vi "Initialize.vi"(7 "Serial Configuration":T1={"Baud Rate"=19200, "Parity"=0, "Data Bits"=8, "Stop Bits"=10, "Flow Control"=2} {"Flow Control" items=["None"=0, "RTS/CTS"=2]; "Stop Bits" items=["1.0"=10]; "Data Bits" items=["8"=8]; "Parity" items=["None"]; "Baud Rate" items=["9600"=9600, "19200"=19200, "38400"=38400]}, 8 "error in (no error)":errorcluster, 9 "Reset (True)":bool=TRUE, 10 "ID Query (True)":bool=TRUE, 11 "VISA resource name":refnum<visa-resource-name>) -> (0 "error out":errorcluster, 3 "VISA resource name out":refnum<visa-resource-name>)   [LabVIEW 2015, in "Voltech PM1000+.lvlib"]
doc: "Establishes communication with the instrument and optionally performs an instrument identification query and/or an instrument reset. It also places the instrument in a default state needed for other instrument driver operations. Therefore, call this VI before calling other instrument driver VIs for this instrument. Generally, you need to call the Initialize VI only once at the beginning of an application."
uses:
  <instrlib>/Voltech PM1000+/Voltech PM1000+.lvlib
panel:
  # "(c) 2008-2009 Voltech Instruments.  ALL RIGHTS RESERVED."
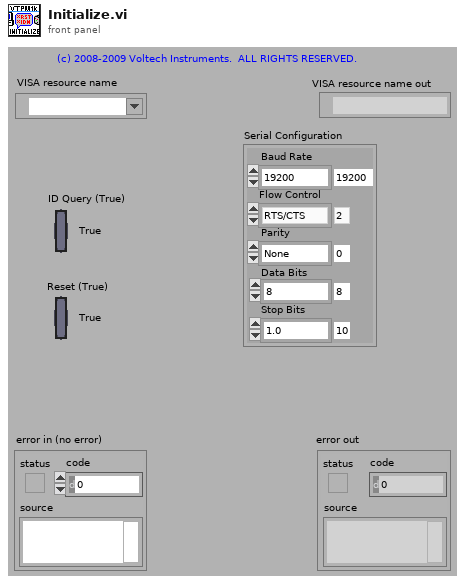
[diagram p1: front panel]
types:
  T1 = cluster{"Baud Rate":u32, "Parity":u16, "Data Bits":u16, "Stop Bits":u16, "Flow Control":u16}
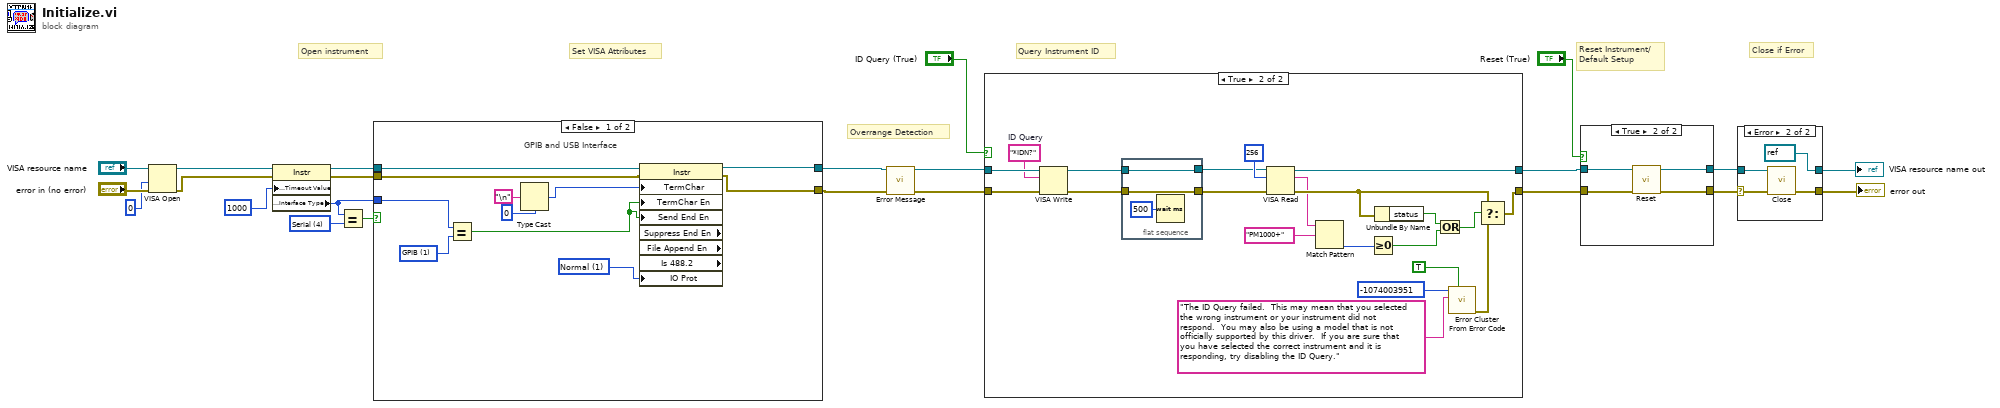
[diagram p0: block diagram]
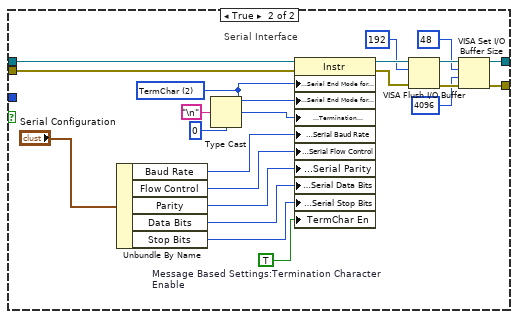
[diagram p2: hidden frame]
diagram:
  w15 = u16 4 items=["GPIB"=1, "Serial"=4, "USB"=7] ("Interface Information:Interface Type")
  # "Overrange Detection"
  # "Set VISA Attributes"
  # "Close if Error"
  # "Query Instrument ID"
  # "Reset Instrument/\nDefault Setup"
  # "Open instrument"
  n1 = VISA Open(access mode=u32 0, error in (no error)="error in (no error)", VISA resource name="VISA resource name") -> (VISA resource name=w8:refnum<visa-resource-name>, error out=w7:errorcluster)  [unwired: 2 in]
  n2 = property class="Instr"(reference=w8, error in=w7, "General Settings:Timeout Value"=u32 1000) -> (reference out=w18:refnum<visa-resource-name>, error out=w17:errorcluster, "Interface Information:Interface Type"=w9:u16)
  n3 = Equal?(x=w9, y=w15) -> (x = y?=w16:bool)
  n4 = case shown="False" w16 {
    tunnel: [w32 w53] -> w6
    tunnel: [w31 w50] -> w3
    tunnel: w18 -> [w34 w55]
    tunnel: w17 -> [w33 w56]
    tunnel: w9 -> [w25 _]
    frame False {
      w26 = u16 1 items=["GPIB"=1, "Serial"=4, "USB"=7] ("Interface Information:Interface Type")
      w27 = u16 1 items=["Normal"=1, "VXI/FDC"=2, "GPIB/HS488"=3, "Serial-TCPIP-USB/488 Strings"=4, "USBTMC/Vendor-Specific"=5] ("Message Based Settings:IO Protocol")
      # "GPIB and USB Interface"
      n5 = Equal?(x=w25, y=w26) -> (x = y?=w24:bool)
      n6 = Type Cast(type=u8 0, x="\n" ("Line Feed Constant")) -> (*(type *) &x=w28:u8)
      n7 = property class="Instr" props=["TermChar", "TermChar En", "Send End En", "Suppress End En", "File Append En", "Is 488.2", "IO Prot"](reference=w34, error in=w33, "TermChar"=w28, "TermChar En"=w24, "Send End En"=w24, "IO Prot"=w27) -> (reference out=w32:refnum<visa-resource-name>, error out=w31:errorcluster)  [unwired: 3 out]
    }
    frame True {
      w43 = u16 2 items=["None", "LastBit", "TermChar"] ("Serial Settings:Serial End Mode for Reads")
      w35 = TRUE  # Message Based Settings:Termination Character Enable
      # "Serial Interface"
      n8 = Unbundle By Name("Serial Configuration") -> ("Baud Rate"=w41:u32, "Flow Control"=w37:u16, "Parity"=w39:u16, "Data Bits"=w40:u16, "Stop Bits"=w36:u16)
      n9 = Type Cast(type=u8 0, x="\n" ("Line Feed Constant")) -> (*(type *) &x=w42:u8)
      n10 = property class="Instr"(reference=w55, error in=w56, "Serial Settings:Serial End Mode for Reads"=w43, "Serial Settings:Serial End Mode for Writes"=w43, "Message Based Settings:Termination Character"=w42, "Serial Settings:Serial Baud Rate"=w41, "Serial Settings:Serial Flow Control"=w37, "Serial Settings:Serial Parity"=w39, "Serial Settings:Serial Data Bits"=w40, "Serial Settings:Serial Stop Bits"=w36, "TermChar En"=w35) -> (reference out=w49:refnum<visa-resource-name>, error out=w52:errorcluster)
      n11 = VISA Flush I/O Buffer(VISA resource name=w49, mask (16)=u16 192, error in (no error)=w52) -> (VISA resource name out=w54:refnum<visa-resource-name>, error out=w51:errorcluster)
      n12 = VISA Set I/O Buffer Size(VISA resource name=w54, mask (16)=u16 48, size (4096)=u32 4096 ("size (0)"), error in (no error)=w51) -> (VISA resource name out=w53:refnum<visa-resource-name>, error out=w50:errorcluster)
    }
  }
  n13 = call <instrlib>:"Error Message.vi"("VISA resource name"=w6, "error in (no error)"=w3) -> ("VISA resource name out"=w4:refnum<visa-resource-name>, "error out"=w5:errorcluster)  [unwired: 12 in]
  n14 = case shown="True" "ID Query (True)" {
    tunnel: [w57 w79] -> w1
    tunnel: [w58 w76] -> w2
    tunnel: w4 -> [w58 w77]
    tunnel: w5 -> [w57 w78]
    frame False {
    }
    frame True {
      w73 = "*IDN?"  # ID Query
      n15 = VISA Write(VISA resource name=w77, write buffer=w73, error in (no error)=w78) -> (VISA resource name out=w62:refnum<visa-resource-name>, error out=w60:errorcluster)  [unwired: 1 out]
      n16 = flat-sequence {
        tunnel: [w81] -> w61
        tunnel: w62 -> [w81]
        tunnel: [w80] -> w59
        tunnel: w60 -> [w80]
        frame #0 {
          n17 = Wait (ms)(milliseconds to wait=500) -> ()  [unwired: 1 out]
        }
      }
      n18 = VISA Read(VISA resource name=w61, byte count=u32 256, error in (no error)=w59) -> (VISA resource name out=w76:refnum<visa-resource-name>, read buffer=w63:string, error out=w67:errorcluster)  [unwired: 1 out]
      n19 = Match Pattern(string=w63, regular expression="PM1000+") -> (offset past match=w68:i32)  [unwired: 1 in, 3 out]
      n20 = Greater Or Equal To 0?(x=w68) -> (x >= 0?=w65:bool)
      n21 = Unbundle By Name(w67) -> ("status"=w66:bool)
      n22 = Or(x=w66, y=w65) -> (x .or. y?=w64:bool)
      n23 = call <vilib>:"Error Cluster From Error Code.vi"("show call chain? (False)"=TRUE, "error message (\"\")"="The ID Query failed.  This may mean that you selected the wrong instrument or your instrument did not respond.  You may also be using a model that is not officially supported by this driver.  If you are sure that you have selected the correct instrument and it is responding, try disabling the ID Query." ("Source (VI Name)"), "error code (0)"=-1074003951 ("Code")) -> ("error out"=w72:errorcluster)  [unwired: 6 in]
      n24 = Select(t=w67, s=w64, f=w72) -> (s? t:f=w79:errorcluster)
    }
  }
  n25 = case shown="True" "Reset (True)" {
    tunnel: w1 -> [w83 w85]
    tunnel: [w83 w88] -> w10
    tunnel: w2 -> [w84 w86]
    tunnel: [w84 w87] -> w11
    frame False {
    }
    frame True {
      n26 = call <instrlib>:"Reset.vi"("error in (no error)"=w85, "VISA resource name"=w86) -> ("error out"=w88:errorcluster, "VISA resource name out"=w87:refnum<visa-resource-name>)  [unwired: 8 in]
    }
  }
  n27 = case shown="Error" w10 {
    selector: w10 -> [w89 w92]
    tunnel: w11 -> [w90 w93]
    tunnel: [w90 refnum<visa-resource-name> refnum ("VISA resource name out")] -> w13
    tunnel: [w89 w94] -> w12
    frame No Error {
    }
    frame Error {
      n28 = call <instrlib>:"Close.vi"("error in (no error)"=w92, "VISA resource name"=w93) -> ("error out"=w94:errorcluster)  [unwired: 9 in]
    }
  }
  "VISA resource name out" <- w13
  "error out" <- w12
